vi "New QControl Info.vi"(8 "error in (no error)":errorcluster) -> (0 "error out":errorcluster, 1 "CreatorComplete Event":refnum<user-event>, 2 "StatueUpdate Event":refnum<user-event>, 3 "New QControl Info":refnum<data-value>)   [LabVIEW 2020, in "New QControl Info.lvclass"]
uses:
  New QControl Info.lvclass
  New QControl Info.lvclass/New QControl Info.ctl
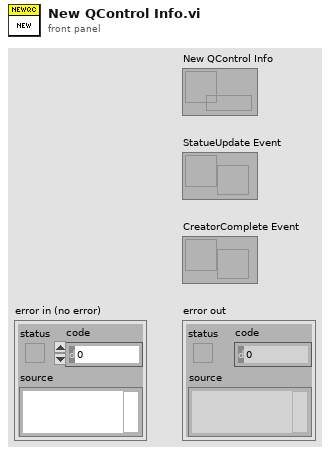
[diagram p1: front panel]
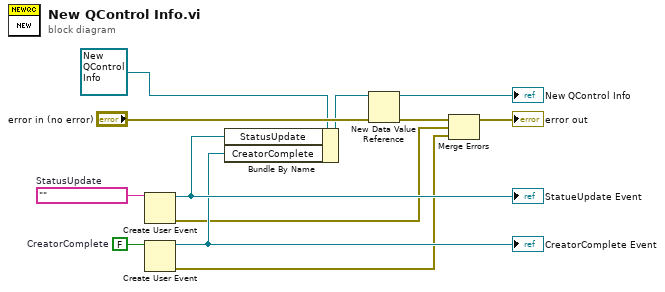
[diagram p0: block diagram]
diagram:
  w9 = FALSE  # CreatorComplete
  w8 = ""  # StatusUpdate
  n1 = Create User Event(user event datatype=w8) -> (user event=w7:refnum<user-event>, error out=w2:errorcluster)  [unwired: 1 in]
  "StatueUpdate Event" <- w7
  n2 = Create User Event(user event datatype=w9) -> (user event=w6:refnum<user-event>, error out=w1:errorcluster)  [unwired: 1 in]
  "CreatorComplete Event" <- w6
  n3 = Bundle By Name(cluster=refnum<class "New QControl Info.lvclass"> refnum ("New QControl Info in"), "StatusUpdate"=w7, "CreatorComplete"=w6) -> (w4:refnum<class "New QControl Info.lvclass">)
  n4 = New Data Value Reference(data value=w4, error in="error in (no error)") -> (data value reference=→"New QControl Info":refnum<data-value>, error out=w10:errorcluster)
  n5 = Merge Errors(w10, w2, w1) -> (→"error out":errorcluster)
